vi "Formic Princess.vi"(8 "error in (no error)":errorcluster, 9 "SelfID":i32, 10 "Map":i32[](array[numeric]), 11 "Mother in":refnum<class "Formics.lvclass">) -> (0 "error out":errorcluster, 1 "Direction":T1, 2 "Action":T2, 3 "Mother out":refnum<class "Formics.lvclass">, 4 "Replicated Class":refnum<class "Formics.lvclass">)   [LabVIEW 2015, in "Formics.lvclass"]
uses:
  Formics.lvclass
  Type Defs/Action Enum.ctl
  Type Defs/Direction Enum.ctl
  Formics.lvclass/Formics.ctl
  SquareStatus.ctl
  Queen Bee Steps.ctl
  Formic Types.ctl
  Square/Square.lvclass
panel:
  in  "Protectors":i32[](array[numeric])=[2, 6]
  out "Kam?":bool
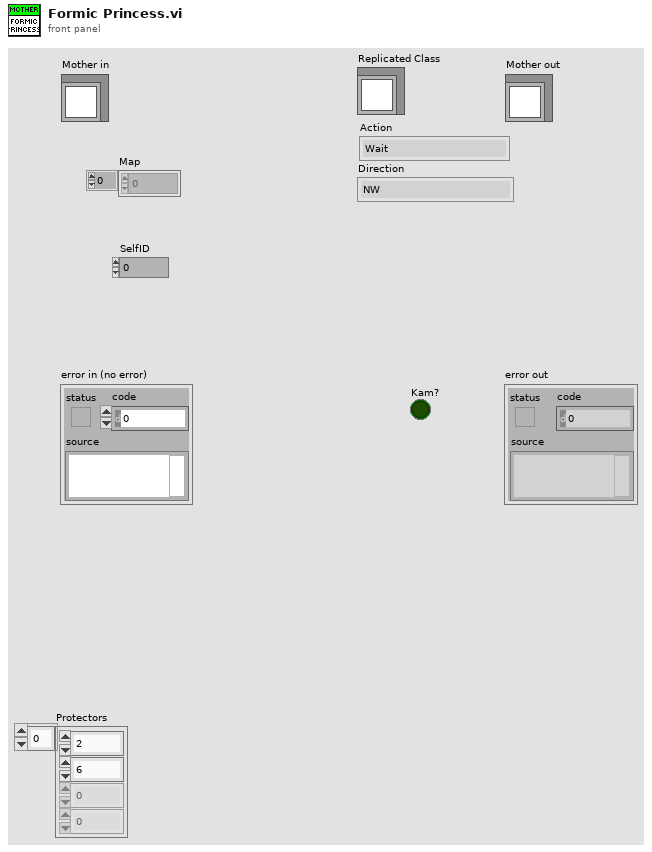
[diagram p1: front panel]
types:
  T1 = typedef "Square.lvclass/Direction Enum.ctl" = enum16{"NW", "N", "NE", "E", "SE", "S", "SW", "W"}
  T2 = typedef "Square.lvclass/Action Enum.ctl" = enum16{"Wait", "Move", "Attack", "Replicate"}
  T3 = enum16{"Queen", "Daughter", "Kamikazee", "Coward", "Migrate", "Line Up"}
  T4 = typedef "Formics.lvclass/Formic Types.ctl" = enum16{"Queen Bee", "Protector Bee", "Daughter Bee", "Worker Bee", "Coward"}
  T5 = typedef "Formics.lvclass/SquareStatus.ctl" = cluster{"ID":i32, "Heartbeat":bool}
  T6 = typedef "Formics.lvclass/SquareStatus DVR.ctl" = refnum<data-value>
  T7 = typedef "Formics.lvclass/Queen Bee Steps.ctl" = enum16{"Attack?", "Migrate?", "Kamikaze?", "Protect?", "Procreate?", "Build Army"}
  T8 = typedef "Formics.lvclass/Kamikaze DVR.ctl" = refnum<data-value>
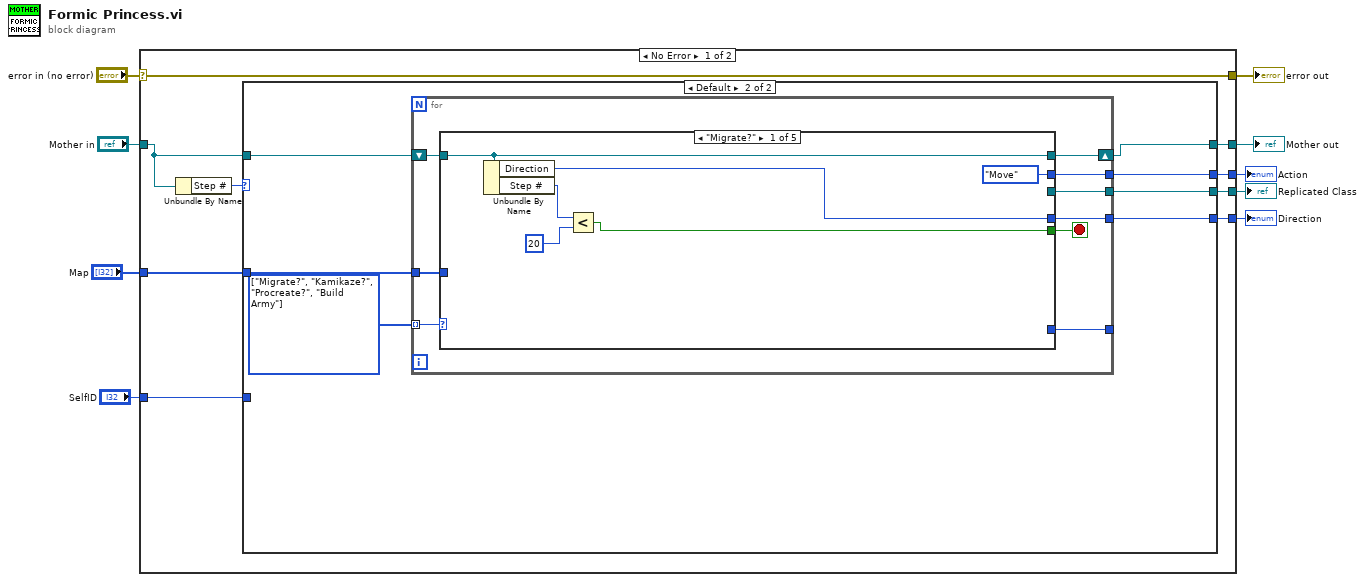
[diagram p0: block diagram]
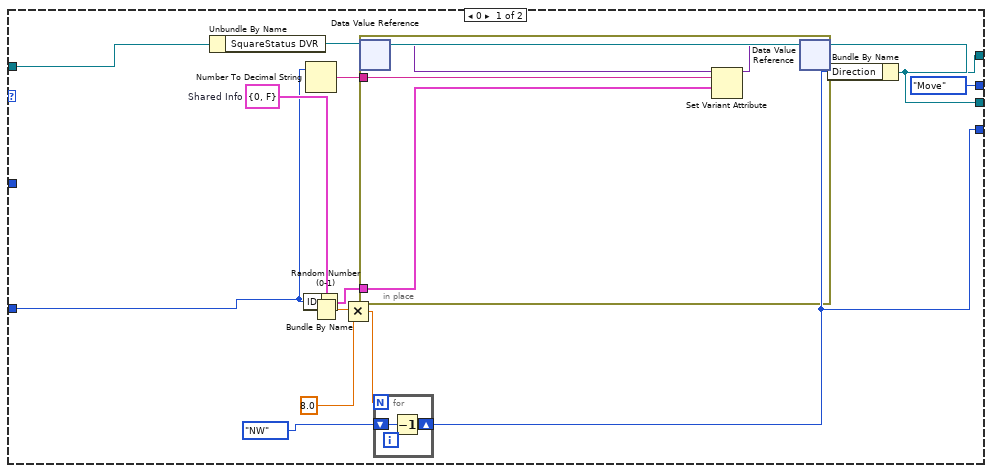
[diagram p2: hidden frame]
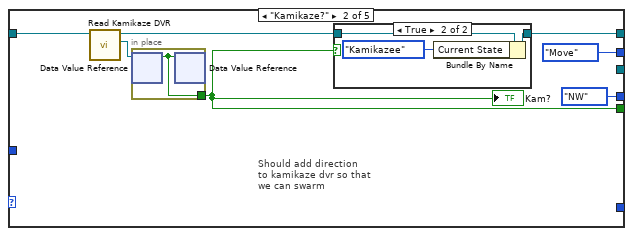
[diagram p3: hidden frame]
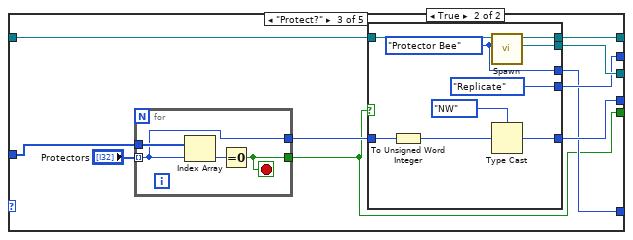
[diagram p5: hidden frame]
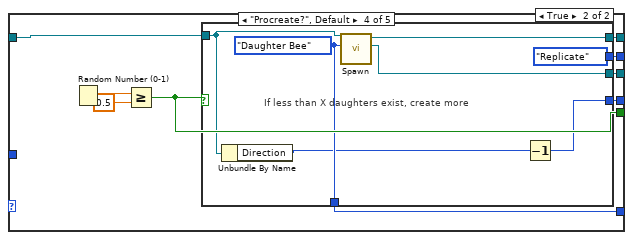
[diagram p7: hidden frame]
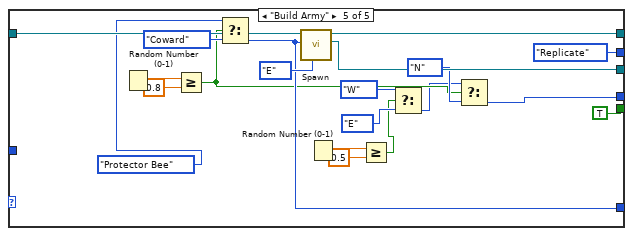
[diagram p9: hidden frame]
diagram:
  n1 = case shown="No Error" "error in (no error)" {
    selector: "error in (no error)" -> [w18 w134]
    tunnel: [w18 w134] -> w8
    tunnel: [w17 w133] -> w6
    tunnel: "Mother in" -> [w16 w133]
    tunnel: "SelfID" -> [w14 _]
    tunnel: "Map" -> [w13 _]
    tunnel: [w12 _] -> w3
    tunnel: [w11 _] -> w2
    tunnel: [w10 _] -> w1
    frame No Error {
      n2 = Unbundle By Name(w16) -> ("Step #"=w15:i32)
      n3 = case shown="Default" w15 {
        tunnel: w16 -> [w30 w44]
        tunnel: [w19 w43] -> w17
        tunnel: w14 -> [w22 _]
        tunnel: w13 -> [_ w41]
        tunnel: [Action_Enum."Move" ("Action") w40] -> w12
        tunnel: [w21 w39] -> w11
        tunnel: [w19 w38] -> w10
        frame 0 {
          w29 = T5 {"ID"=0, "Heartbeat"=FALSE}  # Shared Info
          n4 = Unbundle By Name(w30) -> ("SquareStatus DVR"=w31:T6)
          n5 = Bundle By Name(cluster=w29, "ID"=w22) -> (w27:T5)
          n6 = Number To Decimal String(number=w22) -> (decimal integer string=w28:string)  [unwired: 1 in]
          n7 = Random Number (0-1)() -> (number: 0 to 1=w23:dbl)
          n8 = Multiply(x=w23, y=8.0) -> (x*y=w25:dbl)
          n9 = in-place {
            in-place-border: w28 -> [w35]
            in-place-border: w27 -> [w34]
            n10 = in-place-dvr #1(w31) -> (w37:variant)  [unwired: 1 out]
            n11 = Set Variant Attribute(Variant=w37, name=w35, value=w34) -> (Variant out=w36:variant)  [unwired: 1 in, 2 out]
            n12 = in-place-dvr #1(w36) -> ()  [unwired: 2 out]
          }
          n13 = for {
            N: w25 -> [_]
            shift-right: [w32] -> w21
            shift-left: Direction_Enum."NW" ("Direction") -> [w33]
            n14 = Decrement(x=w33) -> (x-1=w32:T1)
          }
          n15 = Bundle By Name(cluster=w30, "Direction"=w21) -> (w19:refnum<class "Formics.lvclass">)
        }
        frame Default {
          w42 = T7[] [enum."Migrate?", enum."Kamikaze?", enum."Procreate?", enum."Build Army"] items=["Attack?", "Migrate?", "Kamikaze?", "Protect?", "Procreate?", "Build Army"]
          n16 = for {
            tunnel: w41 -> [w51]
            shift-right: [w52] -> w43
            shift-left: w44 -> [w53]
            tunnel: [w50] -> w40
            tunnel: [w49] -> w39
            tunnel: w42 -> [w48] mode=indexing
            tunnel: [w46] -> w38
            tunnel: [w45] -> _
            stop <- w47 stop-if-true
            n17 = case shown="\"Migrate?\"" w48 {
              tunnel: w53 -> [w59 w66 w81 w99 w132]
              tunnel: [w59 w63 w80 w102 w129] -> w52
              tunnel: w51 -> [_ _ w77 _ _]
              tunnel: [Action_Enum."Move" ("Action") Action_Enum."Move" ("Action") w78 w104 Action_Enum."Replicate" ("Action")] -> w50
              tunnel: [w54 Direction_Enum."NW" ("Direction") w74 w103 w120] -> w49
              tunnel: [w56 w61 w72 w96 TRUE ("Enemy Found?")] -> w47
              tunnel: [_ _ w79 w101 w128] -> w46
              tunnel: [_ _ w73 w100 w122] -> w45
              frame "Migrate?" {
                n18 = Unbundle By Name(w59) -> ("Direction"=w54:i32, "Step #"=w58:i32)
                n19 = Less?(x=w58, y=20 ("# Steps")) -> (x < y?=w56:bool)
              }
              frame "Kamikaze?" {
                # "Should add direction\nto kamikaze dvr so that\nwe can swarm"
                n20 = call "Read Kamikaze DVR.vi"("Mother in"=w66) -> ("Kamikaze DVR"=w64:T8, "Mother out"=w62:refnum<class "Formics.lvclass">)  [unwired: 8 in, 1 out]
                n21 = in-place {
                  in-place-border: [w71] -> w61
                  n22 = in-place-dvr #2(w64) -> (w71:bool)  [unwired: 1 out]
                  n23 = in-place-dvr #2(w71) -> ()  [unwired: 2 out]
                }
                "Kam?" <- w61
                n24 = case shown="True" w61 {
                  tunnel: [w67 w70] -> w63
                  tunnel: w62 -> [w67 w69]
                  frame False {
                  }
                  frame True {
                    n25 = Bundle By Name(cluster=w69, "Current State"=T3."Kamikazee") -> (w70:refnum<class "Formics.lvclass">)
                  }
                }
              }
              frame "Protect?" {
                n26 = for {
                  tunnel: w77 -> [w95]
                  tunnel: [w94] -> w72
                  tunnel: "Protectors" -> [w92] mode=indexing
                  tunnel: [w92] -> w75
                  stop <- w94 stop-if-true
                  n27 = Index Array(array=w95, index=w92) -> (element=w93:i32)
                  n28 = Equal To 0?(x=w93) -> (x = 0?=w94:bool)
                }
                n29 = case shown="True" w72 {
                  tunnel: w81 -> [w82 w91]
                  tunnel: [w82 w90] -> w80
                  tunnel: [_ w89] -> w79
                  tunnel: [_ Action_Enum."Replicate" ("Action")] -> w78
                  tunnel: w75 -> [_ w86]
                  tunnel: [_ w85] -> w74
                  tunnel: [_ w83] -> w73
                  frame False {
                  }
                  frame True {
                    w83 = Formic_Types."Protector Bee"
                    n30 = To Unsigned Word Integer(number=w86) -> (unsigned 16bit integer=w87:u16)
                    n31 = call "Spawn.vi"(10:w83, "Mother in"=w91) -> ("Replicated Class"=w89:refnum<class "Formics.lvclass">, "Mother out"=w90:refnum<class "Formics.lvclass">)  [unwired: 7 in, 1 out]
                    n32 = Type Cast(type=Direction_Enum."NW" ("Direction"), x=w87) -> (*(type *) &x=w85:T1)
                  }
                }
              }
              frame "Procreate?", Default {
                n33 = Random Number (0-1)() -> (number: 0 to 1=w98:dbl)
                n34 = Greater Or Equal?(x=w98, y=0.5) -> (x >= y?=w96:bool)
                n35 = case shown="True" w96 {
                  tunnel: [_ Action_Enum."Replicate" ("Action")] -> w104
                  tunnel: [_ w108] -> w103
                  tunnel: [w105 w111] -> w102
                  tunnel: [_ w110] -> w101
                  tunnel: [_ w109] -> w100
                  tunnel: w99 -> [w105 w107]
                  frame False {
                  }
                  frame True {
                    w109 = Formic_Types."Daughter Bee"
                    # "If less than X daughters exist, create more"
                    n36 = Unbundle By Name(w107) -> ("Direction"=w106:i32)
                    n37 = call "Spawn.vi"(10:w109, "Mother in"=w107) -> ("Replicated Class"=w110:refnum<class "Formics.lvclass">, "Mother out"=w111:refnum<class "Formics.lvclass">)  [unwired: 7 in, 1 out]
                    n38 = Decrement(x=w106) -> (x-1=w108:i32)
                  }
                }
              }
              frame "Build Army" {
                n39 = Random Number (0-1)() -> (number: 0 to 1=w123:dbl)
                n40 = Greater Or Equal?(x=w123, y=0.8) -> (x >= y?=w118:bool)
                n41 = Select(t=Formic_Types."Protector Bee", s=w118, f=Formic_Types."Coward") -> (s? t:f=w122:T4)
                n42 = call "Spawn.vi"("Start Direction"=Direction_Enum."E", 10:w122, "Mother in"=w132) -> ("Replicated Class"=w128:refnum<class "Formics.lvclass">, "Mother out"=w129:refnum<class "Formics.lvclass">)  [unwired: 6 in, 1 out]
                n43 = Random Number (0-1)() -> (number: 0 to 1=w117:dbl)
                n44 = Greater Or Equal?(x=w117, y=0.5) -> (x >= y?=w113:bool)
                n45 = Select(t=Direction_Enum."W", s=w113, f=Direction_Enum."E" ("Direction")) -> (s? t:f=w115:T1)
                n46 = Select(t=w115, s=w118, f=Direction_Enum."N" ("Direction")) -> (s? t:f=w120:T1)
              }
            }
          }
        }
      }
    }
    frame Error {
    }
  }
  "error out" <- w8
  "Mother out" <- w6
  "Action" <- w3
  "Direction" <- w2
  "Replicated Class" <- w1
